vi "Tri-Tri intersection test.vi"(2 "Triangle 2":T1, 3 "Triangle 1":T1) -> (0 "Intersection point":sgl[](array[numeric]), 1 "Intersection":bool)   [LabVIEW 2014]
uses:
  Typedefs/Triangle.ctl
  Subroutines/Point-in-Tri test.vi
  Subroutines/Edge-Plane intersection test.vi
  Subroutines/Dot product.vi
panel:
  # "PN 12/01/2015"
  # "Vertices"
  # "Edges"
  # "Unit normal"
  # "Edge unit normals"
  # "Vertices"
  # "Edges"
  # "Unit normal"
  # "Edge unit normals"
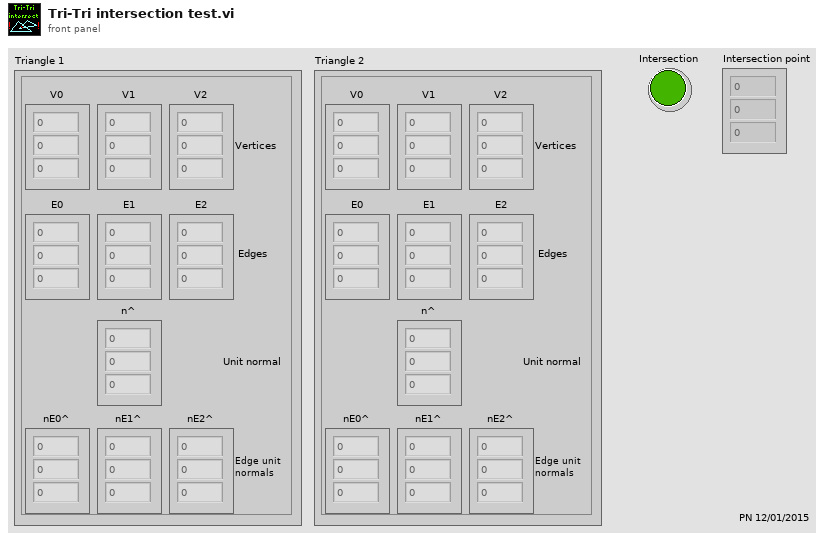
[diagram p1: front panel]
types:
  T1 = typedef "Triangle.ctl" = cluster{"V0":sgl[], "V1":sgl[], "V2":sgl[], "E0":sgl[], "E1":sgl[], "E2":sgl[], "n^":sgl[], "nE0^":sgl[], "nE1^":sgl[], "nE2^":sgl[]}
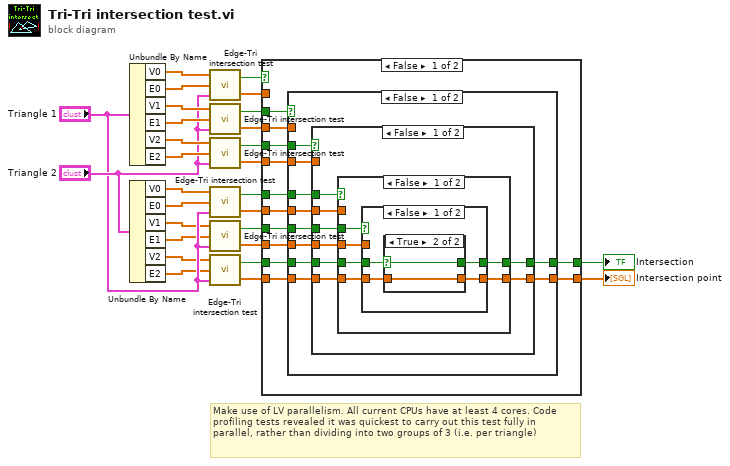
[diagram p0: block diagram]
diagram:
  # "Make use of LV parallelism. All current CPUs have at least 4 cores. Code profiling tests revealed it was quickest to carry out this test fully in parallel, rather than dividing into two groups of 3 (i.e. per triangle)"
  n1 = Unbundle By Name("Triangle 1") -> ("V0"=w28:sgl[], "E0"=w27:sgl[], "V1"=w26:sgl[], "E1"=w25:sgl[], "V2"=w24:sgl[], "E2"=w23:sgl[])
  n2 = Unbundle By Name("Triangle 2") -> ("V0"=w9:sgl[], "E0"=w10:sgl[], "V1"=w11:sgl[], "E1"=w12:sgl[], "V2"=w13:sgl[], "E2"=w14:sgl[])
  n3 = call "Edge-Tri intersection test.vi"("Triangle"="Triangle 2", "Edge vector (not unit)"=w27, "Edge start point"=w28) -> ("Intersection point"=w21:sgl[], "Intersection"=w22:bool)
  n4 = call "Edge-Tri intersection test.vi"("Triangle"="Triangle 2", "Edge vector (not unit)"=w25, "Edge start point"=w26) -> ("Intersection point"=w18:sgl[], "Intersection"=w20:bool)
  n5 = call "Edge-Tri intersection test.vi"("Triangle"="Triangle 2", "Edge vector (not unit)"=w23, "Edge start point"=w24) -> ("Intersection point"=w17:sgl[], "Intersection"=w19:bool)
  n6 = call "Edge-Tri intersection test.vi"("Triangle"="Triangle 1", "Edge vector (not unit)"=w10, "Edge start point"=w9) -> ("Intersection point"=w7:sgl[], "Intersection"=w8:bool)
  n7 = call "Edge-Tri intersection test.vi"("Triangle"="Triangle 1", "Edge vector (not unit)"=w12, "Edge start point"=w11) -> ("Intersection point"=w5:sgl[], "Intersection"=w6:bool)
  n8 = call "Edge-Tri intersection test.vi"("Triangle"="Triangle 1", "Edge vector (not unit)"=w14, "Edge start point"=w13) -> ("Intersection point"=w3:sgl[], "Intersection"=w4:bool)
  n9 = case shown="False" w22 {
    selector: w22 -> [_ w82]
    tunnel: w21 -> [_ w81]
    tunnel: w20 -> [w40 _]
    tunnel: w19 -> [w39 _]
    tunnel: w18 -> [w38 _]
    tunnel: w17 -> [w37 _]
    tunnel: [w36 w82] -> w2
    tunnel: [w35 w81] -> w1
    tunnel: w8 -> [w34 _]
    tunnel: w7 -> [w33 _]
    tunnel: w6 -> [w32 _]
    tunnel: w5 -> [w31 _]
    tunnel: w4 -> [w30 _]
    tunnel: w3 -> [w29 _]
    frame False {
      n10 = case shown="False" w40 {
        selector: w40 -> [_ w80]
        tunnel: w39 -> [w50 _]
        tunnel: w38 -> [_ w79]
        tunnel: w37 -> [w49 _]
        tunnel: [w48 w80] -> w36
        tunnel: [w47 w79] -> w35
        tunnel: w34 -> [w46 _]
        tunnel: w33 -> [w45 _]
        tunnel: w32 -> [w44 _]
        tunnel: w31 -> [w43 _]
        tunnel: w30 -> [w42 _]
        tunnel: w29 -> [w41 _]
        frame False {
          n11 = case shown="False" w50 {
            selector: w50 -> [_ w78]
            tunnel: w49 -> [_ w77]
            tunnel: [w52 w78] -> w48
            tunnel: [w51 w77] -> w47
            tunnel: w46 -> [w58 _]
            tunnel: w45 -> [w57 _]
            tunnel: w44 -> [w56 _]
            tunnel: w43 -> [w55 _]
            tunnel: w42 -> [w54 _]
            tunnel: w41 -> [w53 _]
            frame False {
              n12 = case shown="False" w58 {
                selector: w58 -> [_ w76]
                tunnel: w57 -> [_ w75]
                tunnel: w56 -> [w64 _]
                tunnel: w55 -> [w63 _]
                tunnel: w54 -> [w62 _]
                tunnel: w53 -> [w61 _]
                tunnel: [w60 w76] -> w52
                tunnel: [w59 w75] -> w51
                frame False {
                  n13 = case shown="False" w64 {
                    selector: w64 -> [_ w74]
                    tunnel: w63 -> [_ w73]
                    tunnel: w62 -> [w68 _]
                    tunnel: w61 -> [w67 _]
                    tunnel: [w66 w74] -> w60
                    tunnel: [w65 w73] -> w59
                    frame False {
                      n14 = case shown="True" w68 {
                        selector: w68 -> [w70 w72]
                        tunnel: w67 -> [w69 w71]
                        tunnel: [w70 w72] -> w66
                        tunnel: [w69 w71] -> w65
                        frame False {
                        }
                        frame True {
                        }
                      }
                    }
                    frame True {
                    }
                  }
                }
                frame True {
                }
              }
            }
            frame True {
            }
          }
        }
        frame True {
        }
      }
    }
    frame True {
    }
  }
  "Intersection" <- w2
  "Intersection point" <- w1
